vi "Send Global Chat.vi"(8 "error in (no error)":errorcluster, 10 "Message":string, 11 "Server in":refnum<class "Server.lvclass">) -> (0 "error out":errorcluster, 3 "Server out":refnum<class "Server.lvclass">)   [LabVIEW 2018, in "Server.lvlib" / "Server.lvclass"]
uses:
  Server.lvclass
  Server.lvclass/Server.ctl
  Chat Room Model/Chat Room Model Messages/Update Message Msg/Update Message Msg.lvclass/Update Message Msg.ctl
  <vilib>/ActorFramework/Message Enqueuer/Message Enqueuer.lvclass/Message Enqueuer.ctl
  <vilib>/ActorFramework/Message Enqueuer/Enqueue.vi
  Chat Room Model/Chat Room Model Messages/Update Message Msg/Update Message Msg.lvclass
  C:/Program Files (x86)/National Instruments/LabVIEW 2018/vi.lib/ActorFramework/Message/Message.lvclass
  <vilib>/ActorFramework/Message Priority Queue/Priority Enqueue.vi
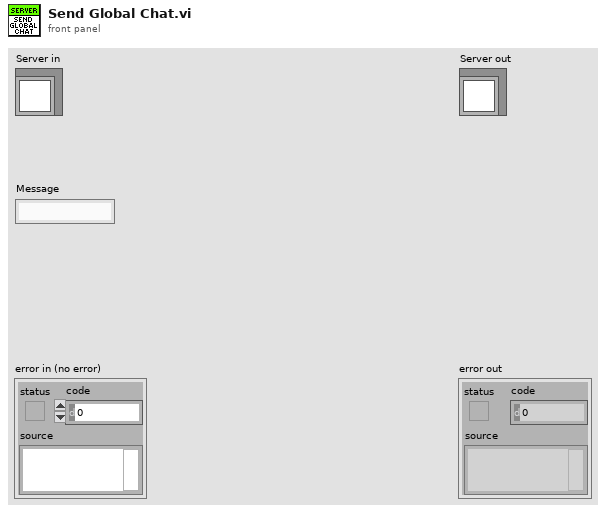
[diagram p1: front panel]
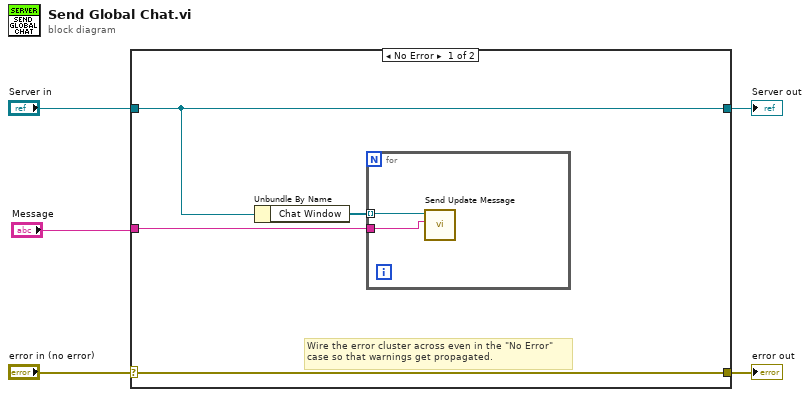
[diagram p0: block diagram]
diagram:
  n1 = case shown="No Error" "error in (no error)" {
    selector: "error in (no error)" -> [w9 w13]
    tunnel: [w9 w13] -> w4
    tunnel: [w8 w12] -> w2
    tunnel: "Server in" -> [w8 w12]
    tunnel: "Message" -> [w6 _]
    frame No Error {
      # "Wire the error cluster across even in the \"No Error\"\ncase so that warnings get propagated."
      n2 = Unbundle By Name(w8) -> ("Chat Window"=w7:refnum<class "Message Enqueuer.lvclass">[])
      n3 = for {
        tunnel: w7 -> [w11] mode=indexing
        tunnel: w6 -> [w10]
        n4 = call "Send Update Message.vi"("Message"=w10, "Message Enqueuer"=w11) -> ()  [unwired: 8 in, 2 out]
      }
    }
    frame Error {
    }
  }
  "error out" <- w4
  "Server out" <- w2
